vi "Database Process.vi"(8 "error in (no error)":errorcluster, 11 "View Model":T3) -> (0 "error out":errorcluster)   [LabVIEW 2017]
doc: "This is separate UI for full access to the data records.\n[Covers: SD6]"
uses:
  View Model/Controls/View Model.ctl
  View Model/Controls/Shared Model.ctl
  Error Handler/Controls/Error Model.ctl
  Error Handler/Controls/Error Message.ctl
  Error Handler/Controls/Error Level.ctl
  Controls/Database Model.ctl
  Controls/Database Message.ctl
  Controls/Database Command.ctl
  Controls/Database Overhead.ctl
  Controls/Database Status.ctl
  Controls/Database Record.ctl
  Controls/Database - Rule Record.ctl
  Controller/Controls/CNTRLR - Wash Step.ctl
  Controller/Controls/CNTRLR - Position.ctl
  Controller/Controls/CNTRLR - Model.ctl
  Controller/Controls/CNTRLR - Message.ctl
  Controller/Controls/CNTRLR - Command.ctl
  Controller/Controls/CNTRLR - Overhead.ctl
  Controller/Controls/CNTRLR - State.ctl
panel:
  out "Timing Data 2":dbl
  out "Timing Data":dbl
  in  "Run":bool
  in  "DB Record":T1
  in  "DB Command":T2
  out "DB Records":T1[](array[typedef])
  # "Used for Insert New Data\nUpdate Exist Data or Query\nTiming Data"
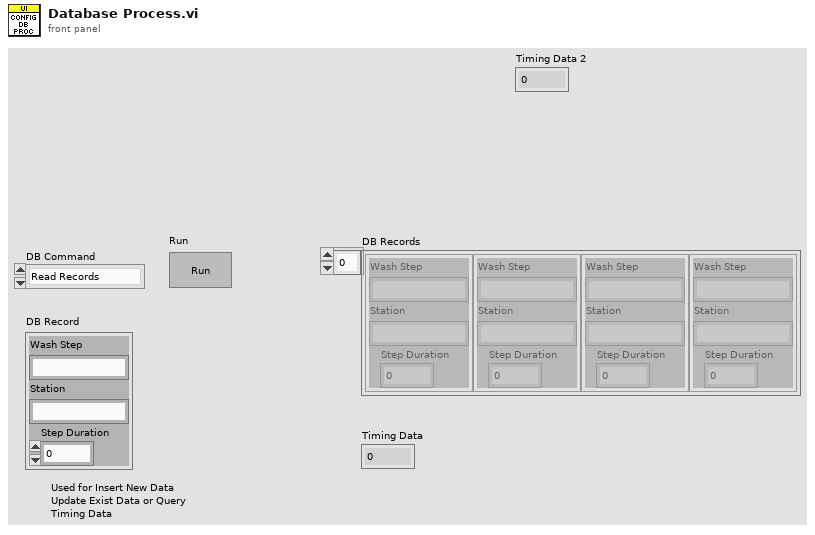
[diagram p1: front panel]
types:
  T1 = typedef "Database Record.ctl" = cluster{"Wash Step":string, "Station":string, "Step Duration":u32}
  T2 = typedef "Database Command.ctl" = enum16{"Read Records", "Query Timing", "Insert New Data", "Update Data"}
  T3 = typedef "View Model.ctl" = cluster{"Shared Model":T4, "Error Model":T5, "DB Model":T6, "CNTRLR Model":T7}
  T4 = typedef "Shared Model.ctl" = cluster{"Stop":refnum<user-event>, "Stop DVR":refnum<data-value>}
  T5 = typedef "Error Model.ctl" = cluster{"Error Message":refnum<user-event>}
  T6 = typedef "Database Model.ctl" = cluster{"DB Message":refnum<user-event>, "DB Overhead DVR":refnum<data-value>}
  T7 = typedef "CNTRLR - Model.ctl" = cluster{"Message":refnum<user-event>, "Overhead DVR":refnum<data-value>, "Wash Entry":refnum<user-event>, "Out of Position":refnum<user-event>}
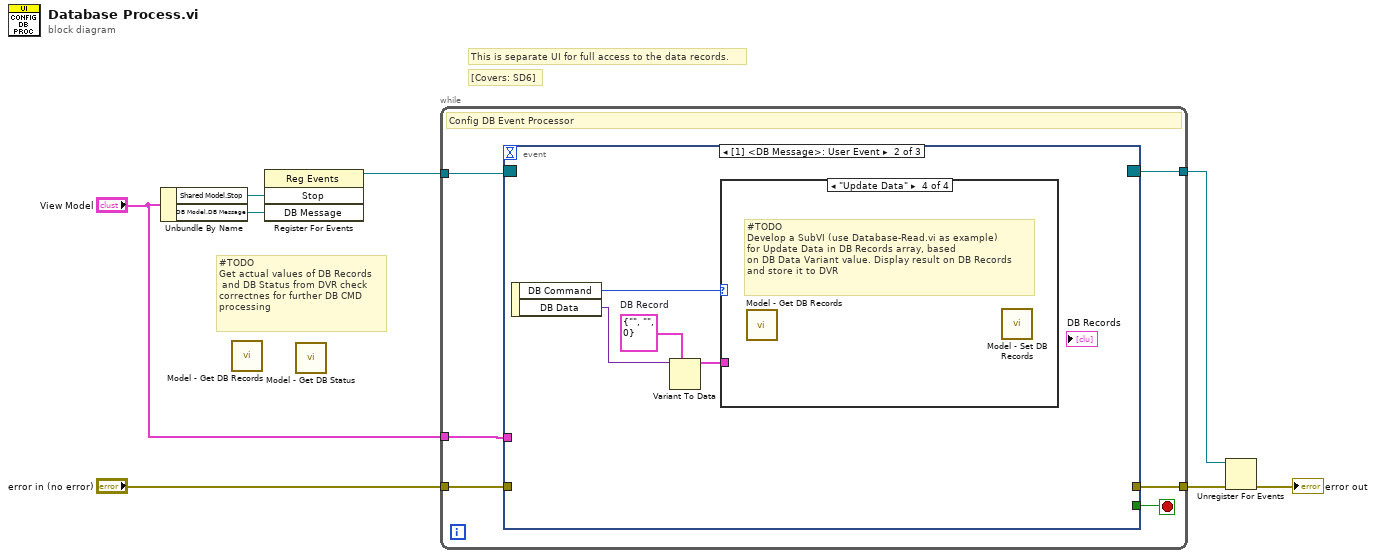
[diagram p0: block diagram]
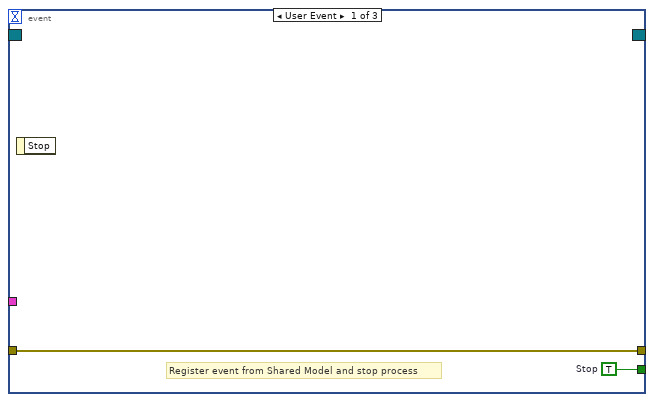
[diagram p2: hidden frame]
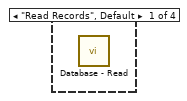
[diagram p3: hidden frame]
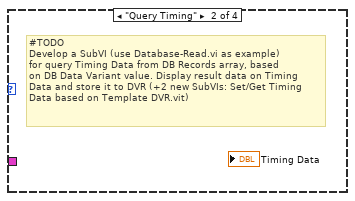
[diagram p4: hidden frame]
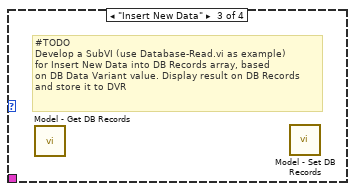
[diagram p5: hidden frame]
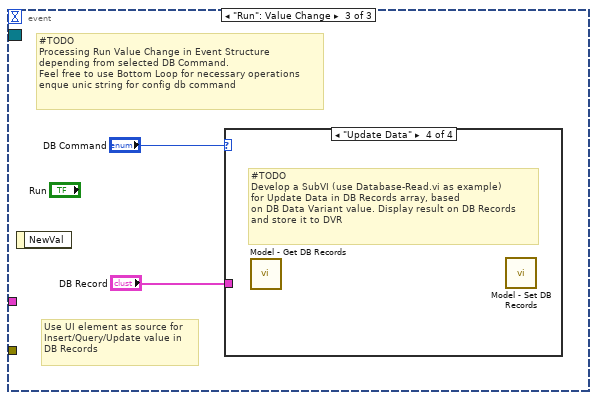
[diagram p6: hidden frame]
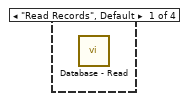
[diagram p7: hidden frame]
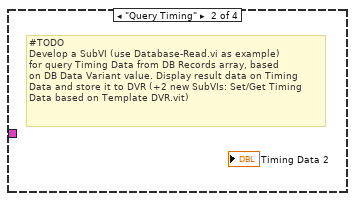
[diagram p8: hidden frame]
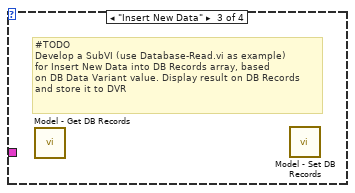
[diagram p9: hidden frame]
diagram:
  # "[Covers: SD6]"
  # "This is separate UI for full access to the data records."
  # "#TODO\nGet actual values of DB Records\n and DB Status from DVR check\ncorrectnes for further DB CMD \nprocessing"
  n1 = Unbundle By Name("View Model") -> ("Shared Model.Stop"=w8:refnum<user-event>, "DB Model.DB Message"=w3:refnum<user-event>)
  n2 = call "Model - Get DB Records.vi"() -> ()  [unwired: 9 in, 3 out]
  n3 = register-events(w8, w3) -> (reference out=w7:refnum<event-registration>)  [unwired: 2 in, 1 out]
  n4 = call "Model - Get DB Status.vi"() -> ()  [unwired: 9 in, 3 out]
  n5 = while {
    tunnel: w7 -> [w14]
    tunnel: "error in (no error)" -> [w13]
    tunnel: [w12] -> w5
    tunnel: [w10] -> w6
    tunnel: "View Model" -> [w9]
    stop <- w11 stop-if-true
    # "Config DB Event Processor"
    n6 = event shown="[1] <DB Message>: User Event" {
      selector: w14 -> [_ _ _]
      dyn-events: [_ _ _] -> w10
      timeout: _ -> [_ _ _]
      tunnel: w13 -> [w15 _ _]
      tunnel: [w15 _ _] -> w12
      tunnel: [w16 _ _] -> w11
      tunnel: w9 -> [_ _ _]
      event User Event {
        w16 = TRUE  # Stop
        # "Register event from Shared Model and stop process"
        n7 = event-data() -> ()  [unwired: 1 in, 1 out]
      }
      event User Event {
        w19 = T1 {"Wash Step"="", "Station"="", "Step Duration"=0}  # DB Record
        n8 = event-data() -> ("DB Command"=w20:T2, "DB Data"=w18:variant)  [unwired: 1 in]
        n9 = Variant To Data(type=w19, Variant=w18) -> (data=w17:T1)  [unwired: 1 in, 1 out]
        n10 = case shown="\"Update Data\"" w20 {
          tunnel: w17 -> [_ _ _ _]
          frame "Read Records", Default {
            n11 = call "Database - Read.vi"() -> ()  [unwired: 10 in, 2 out]
          }
          frame "Query Timing" {
            # "#TODO\nDevelop a SubVI (use Database-Read.vi as example)\nfor query Timing Data from DB Records array, based\non DB Data Variant value. Display result data on Timing\nData and store it to DVR (+2 new SubVIs: Set/Get Timing\nData based on Template DVR.vit)"
          }
          frame "Insert New Data" {
            # "#TODO\nDevelop a SubVI (use Database-Read.vi as example)\nfor Insert New Data into DB Records array, based\non DB Data Variant value. Display result on DB Records\nand store it to DVR"
            n12 = call "Model - Get DB Records.vi"() -> ()  [unwired: 9 in, 3 out]
            n13 = call "Model - Set DB Records.vi"() -> ()  [unwired: 10 in, 2 out]
          }
          frame "Update Data" {
            # "#TODO\nDevelop a SubVI (use Database-Read.vi as example)\nfor Update Data in DB Records array, based\non DB Data Variant value. Display result on DB Records\nand store it to DVR"
            n14 = call "Model - Get DB Records.vi"() -> ()  [unwired: 9 in, 3 out]
            n15 = call "Model - Set DB Records.vi"() -> ()  [unwired: 10 in, 2 out]
          }
        }
      }
      event "Run": Value Change {
        # "Use UI element as source for\nInsert/Query/Update value in\nDB Records"
        # "#TODO\nProcessing Run Value Change in Event Structure\ndepending from selected DB Command.\nFeel free to use Bottom Loop for necessary operations\nenque unic string for config db command"
        n16 = event-data() -> ()  [unwired: 1 in, 1 out]
        n17 = case shown="\"Update Data\"" "DB Command" {
          tunnel: "DB Record" -> [_ _ _ _]
          frame "Read Records", Default {
            n18 = call "Database - Read.vi"() -> ()  [unwired: 10 in, 2 out]
          }
          frame "Query Timing" {
            # "#TODO\nDevelop a SubVI (use Database-Read.vi as example)\nfor query Timing Data from DB Records array, based\non DB Data Variant value. Display result data on Timing\nData and store it to DVR (+2 new SubVIs: Set/Get Timing\nData based on Template DVR.vit)"
          }
          frame "Insert New Data" {
            # "#TODO\nDevelop a SubVI (use Database-Read.vi as example)\nfor Insert New Data into DB Records array, based\non DB Data Variant value. Display result on DB Records\nand store it to DVR"
            n19 = call "Model - Get DB Records.vi"() -> ()  [unwired: 9 in, 3 out]
            n20 = call "Model - Set DB Records.vi"() -> ()  [unwired: 10 in, 2 out]
          }
          frame "Update Data" {
            # "#TODO\nDevelop a SubVI (use Database-Read.vi as example)\nfor Update Data in DB Records array, based\non DB Data Variant value. Display result on DB Records\nand store it to DVR"
            n21 = call "Model - Get DB Records.vi"() -> ()  [unwired: 9 in, 3 out]
            n22 = call "Model - Set DB Records.vi"() -> ()  [unwired: 10 in, 2 out]
          }
        }
      }
    }
  }
  n23 = Unregister For Events(event registration refnum=w6, error in=w5) -> (error out=→"error out":errorcluster)
